vi "Agilent PWM Read Offset Status.vi"(7 "Agilent PWM":T1, 8 "error in (no error)":errorcluster, 11 "VISA Resource Name":refnum<visa-resource-name>) -> (0 "error out":errorcluster, 2 "On/Off":bool, 3 "dup VISA Resource Name":refnum<visa-resource-name>)   [LabVIEW 2011]
doc: "This VI for the HP 8753 is used to read the sweep type.\n\n0 LINEAR FREQ\n1 LOG FREQ\n2 LIST FREQ\n3 CW TIME\n4 POWER SWEEP"
uses:
  TypeDefs/Agilent PWM Instrument Info.ctl
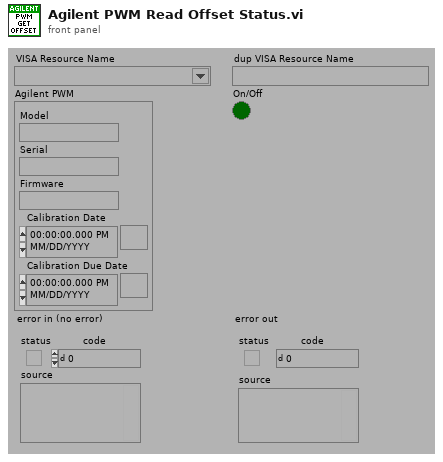
[diagram p1: front panel]
types:
  T1 = typedef "Agilent PWM Instrument Info.ctl" = cluster{"Model":string, "Serial":string, "Firmware":string, "Calibration Date":timestamp, "Calibration Due Date":timestamp}
  T2 = typedef "Agilent PWM Model.ctl" = enum16{"Not Supported", "E4418X", "E4419X", "U2000X"}
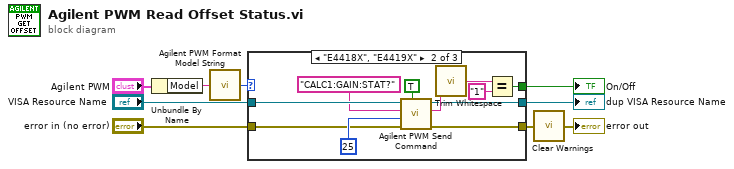
[diagram p0: block diagram]
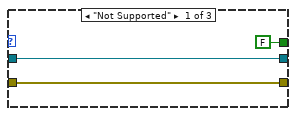
[diagram p2: hidden frame]
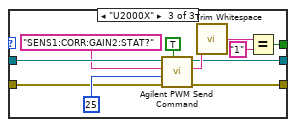
[diagram p3: hidden frame]
diagram:
  n1 = Unbundle By Name("Agilent PWM") -> ("Model"=w7:string)
  n2 = call "Agilent PWM Format Model String.vi"("Model"=w7) -> ("Model"=w6:T2)
  n3 = case shown="\"E4418X\", \"E4419X\"" w6 {
    tunnel: "error in (no error)" -> [w10 w18 w29]
    tunnel: [w10 w17 w28] -> w4
    tunnel: "VISA Resource Name" -> [w11 w16 w27]
    tunnel: [w11 w15 w26] -> w2
    tunnel: [FALSE w14 w25] -> w1
    frame "Not Supported" {
    }
    frame "E4418X", "E4419X" {
      n4 = call "Agilent PWM Send Command.vi"("Read? (F)"=TRUE, "error in (no error)"=w18, "Byte Count"=u32 25, "Command"="CALC1:GAIN:STAT?" ("write buffer"), "VISA Resource Name"=w16) -> ("error out"=w17:errorcluster, "Data Read"=w21:string, "dup VISA Resource Name"=w15:refnum<visa-resource-name>)  [unwired: 4 out]
      n5 = call <vilib>:"Trim Whitespace.vi"("string"=w21) -> ("trimmed string"=w23:string)  [unwired: 1 in]
      n6 = Equal?(x=w23, y="1") -> (x = y?=w14:bool)
    }
    frame "U2000X" {
      n7 = call "Agilent PWM Send Command.vi"("Read? (F)"=TRUE, "error in (no error)"=w29, "Byte Count"=u32 25, "Command"="SENS1:CORR:GAIN2:STAT?" ("write buffer"), "VISA Resource Name"=w27) -> ("error out"=w28:errorcluster, "Data Read"=w32:string, "dup VISA Resource Name"=w26:refnum<visa-resource-name>)  [unwired: 4 out]
      n8 = call <vilib>:"Trim Whitespace.vi"("string"=w32) -> ("trimmed string"=w34:string)  [unwired: 1 in]
      n9 = Equal?(x=w34, y="1") -> (x = y?=w25:bool)
    }
  }
  "dup VISA Resource Name" <- w2
  "On/Off" <- w1
  n10 = call "Clear Warnings.vi"("error in (no error)"=w4) -> ("error out"=→"error out":errorcluster)
